vi "Set port.vi"(8 "error in (no error)":errorcluster, 9 "Value":string, 10 "Puerto":dbl, 11 "Arduino in":refnum<class "Arduino.lvclass">) -> (0 "error out":errorcluster, 3 "Arduino out":refnum<class "Arduino.lvclass">)   [LabVIEW 2020, in "Arduino.lvclass"]
uses:
  Arduino.lvclass
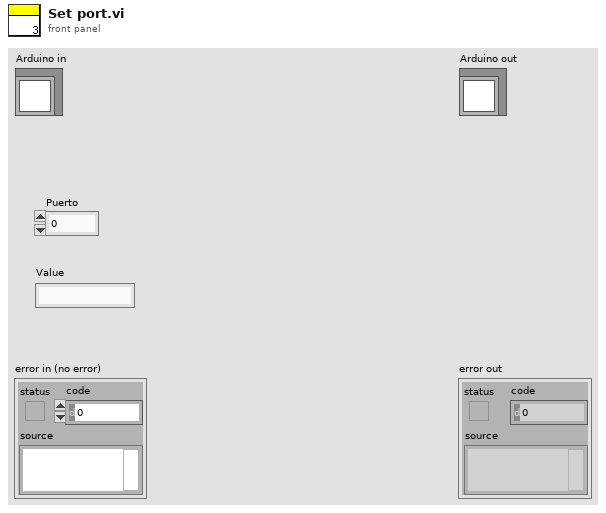
[diagram p1: front panel]
types:
  T1 = typedef "Serial Device.lvclass/serial device brand.ctl" = string
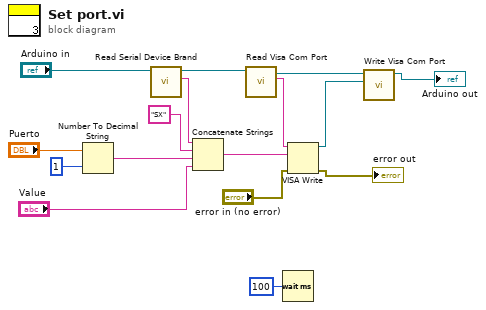
[diagram p0: block diagram]
diagram:
  n1 = Number To Decimal String(number="Puerto", width (-)=i16 1) -> (decimal integer string=w10:string)
  n2 = call-dynamic "Read Serial Device Brand.vi"("Serial Device in"="Arduino in") -> ("Serial Device Brand"=w14:T1, "Serial Device out"=w16:refnum<class "Arduino.lvclass">)  [unwired: 8 in, 1 out]
  n3 = Concatenate Strings(w14, "SX" ("string"), w10, "Value") -> (w8:string)
  n4 = call-dynamic "Read Visa Com Port.vi"("Serial Device in"=w16) -> ("Visa Com Port"=w7:string, "Serial Device out"=w5:refnum<class "Arduino.lvclass">)  [unwired: 8 in, 1 out]
  n5 = Wait (ms)(milliseconds to wait=u32 100) -> ()  [unwired: 1 out]
  n6 = VISA Write(VISA resource name=w7, write buffer=w8, error in (no error)="error in (no error)") -> (VISA resource name out=w6:refnum<visa-resource-name>, error out=→"error out":errorcluster)  [unwired: 1 out]
  n7 = call-dynamic "Write Visa Com Port.vi"("Visa Com Port"=w6, "Serial Device in"=w5) -> ("Serial Device out"=→"Arduino out":refnum<class "Arduino.lvclass">)  [unwired: 8 in, 1 out]
